vi "Intrplt_Get_Dest_Coords.vi"(10 "Dim":i32, 11 "Step":sgl) -> (3 "Coords":sgl[](array[numeric]))   [LabVIEW 2020]
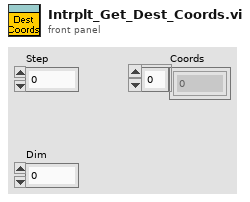
[diagram p1: front panel]
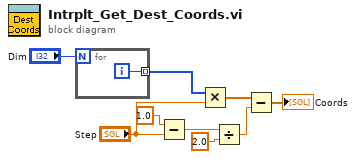
[diagram p0: block diagram]
diagram:
  n1 = for {
    N: "Dim" -> [_]
    tunnel: [w10] -> w2 mode=indexing
    i -> [w10]
  }
  n2 = Subtract(x=sgl 1.0 ("y"), y="Step") -> (x-y=w5:sgl)
  n3 = Multiply(x=w2, y="Step") -> (x*y=w7:sgl[])
  n4 = Divide(x=w5, y=sgl 2.0) -> (x/y=w8:sgl)
  n5 = Subtract(x=w7, y=w8) -> (x-y=→"Coords":sgl[])
